vi "O(tau,tau_0,t_0)_Analytical.vi"(6 "t0":ext, 7 "Harmonic f":ext, 8 "N":i32, 9 "T":ext, 10 "tau_0":ext, 11 "tau":ext) -> (3 "O(tau_tau_0,t_0)":cxt)   [LabVIEW 2019]
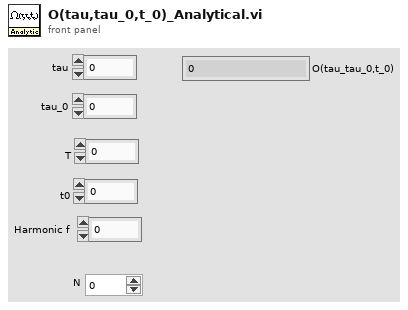
[diagram p1: front panel]
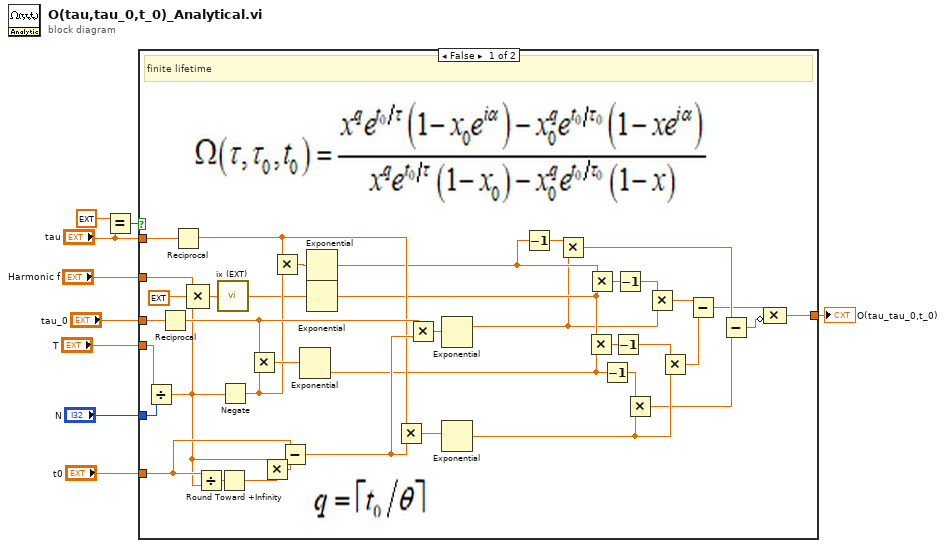
[diagram p0: block diagram]
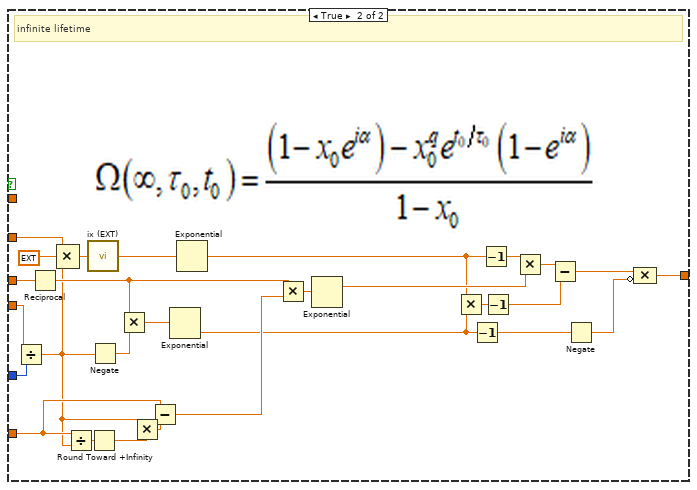
[diagram p2: hidden frame]
diagram:
  n1 = Equal?(x=ext inf, y="tau") -> (x = y?=w2:bool)
  n2 = case shown="False" w2 {
    tunnel: "Harmonic f" -> [w43 w72]
    tunnel: [w47 w75] -> w8
    tunnel: "N" -> [w46 w74]
    tunnel: "T" -> [w45 w73]
    tunnel: "t0" -> [w39 w68]
    tunnel: "tau" -> [w44 _]
    tunnel: "tau_0" -> [w37 w66]
    frame False {
      # "finite lifetime"
      n3 = Divide(x=w45, y=w46) -> (x/y=w10:ext)
      n4 = Reciprocal(x=w37) -> (1/x=w35:ext)
      n5 = Reciprocal(x=w44) -> (1/x=w31:ext)
      n6 = Compound Arithmetic op=MULTIPLY(w43, ext 6.283185307179586477, w10) -> (w42:ext)
      n7 = Divide(x=w39, y=w10) -> (x/y=w41:ext)
      n8 = call "ix (EXT).vi"("x (1)"=w42) -> ("ix"=w28:cxt)
      n9 = Round Toward +Infinity(x=w41) -> (ceil(x): smallest int >= x=w40:ext)
      n10 = Negate(x=w10) -> (-x=w30:ext)
      n11 = Multiply(x=w35, y=w30) -> (x*y=w34:ext)
      n12 = Multiply(x=w10, y=w40) -> (x*y=w38:ext)
      n13 = Multiply(x=w31, y=w30) -> (x*y=w29:ext)
      n14 = Subtract(x=w39, y=w38) -> (x-y=w36:ext)
      n15 = Exponential(1:w34) -> (0:w21:ext)
      n16 = Exponential(1:w29) -> (0:w22:ext)
      n17 = Exponential(1:w28) -> (0:w23:cxt)
      n18 = Multiply(x=w31, y=w36) -> (x*y=w33:ext)
      n19 = Multiply(x=w35, y=w36) -> (x*y=w32:ext)
      n20 = Exponential(1:w32) -> (0:w17:ext)
      n21 = Exponential(1:w33) -> (0:w19:ext)
      n22 = Decrement(x=w22) -> (x-1=w18:ext)
      n23 = Multiply(x=w18, y=w17) -> (x*y=w16:ext)
      n24 = Multiply(x=w23, y=w21) -> (x*y=w26:cxt)
      n25 = Multiply(x=w22, y=w23) -> (x*y=w27:cxt)
      n26 = Decrement(x=w21) -> (x-1=w20:ext)
      n27 = Decrement(x=w26) -> (x-1=w24:cxt)
      n28 = Decrement(x=w27) -> (x-1=w25:cxt)
      n29 = Multiply(x=w20, y=w19) -> (x*y=w15:ext)
      n30 = Multiply(x=w25, y=w17) -> (x*y=w13:cxt)
      n31 = Multiply(x=w24, y=w19) -> (x*y=w12:cxt)
      n32 = Subtract(x=w13, y=w12) -> (x-y=w11:cxt)
      n33 = Subtract(x=w16, y=w15) -> (x-y=w14:ext)
      n34 = Compound Arithmetic op=MULTIPLY(w11, invert w14) -> (w47:cxt)
    }
    frame True {
      # "infinite lifetime"
      n35 = Divide(x=w73, y=w74) -> (x/y=w53:ext)
      n36 = Reciprocal(x=w66) -> (1/x=w64:ext)
      n37 = Compound Arithmetic op=MULTIPLY(w72, ext 6.283185307179586477, w53) -> (w71:ext)
      n38 = Divide(x=w68, y=w53) -> (x/y=w70:ext)
      n39 = call "ix (EXT).vi"("x (1)"=w71) -> ("ix"=w60:cxt)
      n40 = Round Toward +Infinity(x=w70) -> (ceil(x): smallest int >= x=w69:ext)
      n41 = Negate(x=w53) -> (-x=w61:ext)
      n42 = Multiply(x=w64, y=w61) -> (x*y=w63:ext)
      n43 = Multiply(x=w53, y=w69) -> (x*y=w67:ext)
      n44 = Subtract(x=w68, y=w67) -> (x-y=w65:ext)
      n45 = Exponential(1:w63) -> (0:w57:ext)
      n46 = Exponential(1:w60) -> (0:w50:cxt)
      n47 = Multiply(x=w64, y=w65) -> (x*y=w62:ext)
      n48 = Exponential(1:w62) -> (0:w56:ext)
      n49 = Multiply(x=w50, y=w57) -> (x*y=w59:cxt)
      n50 = Decrement(x=w57) -> (x-1=w52:ext)
      n51 = Decrement(x=w50) -> (x-1=w58:cxt)
      n52 = Decrement(x=w59) -> (x-1=w49:cxt)
      n53 = Multiply(x=w58, y=w56) -> (x*y=w55:cxt)
      n54 = Subtract(x=w55, y=w49) -> (x-y=w54:cxt)
      n55 = Negate(x=w52) -> (-x=w51:ext)
      n56 = Compound Arithmetic op=MULTIPLY(w54, invert w51) -> (w75:cxt)
    }
  }
  "O(tau_tau_0,t_0)" <- w8
